vi "Read Relative Calculation.vi"(8 "error in (no error)":errorcluster, 11 "VISA resource name":refnum<visa-resource-name>) -> (0 "error out":errorcluster, 2 "Rel'd Measurement Data":dbl[][](array[numeric]), 3 "VISA resource name out":refnum<visa-resource-name>)   [LabVIEW 2020, in "Keithley 6517.lvlib"]
doc: "Reads the Rel'd measurement data. \n\nRelative (Rel) nulls an offset or subtracts a baseline reading from present and future readings. When a Rel value is established, subsequent readings will be the difference between the actual input and the Rel value.\n\n<B>Displayed (Rel'ed) Reading = Actual Input - Rel Value</B>\n\n<B>Note:</B>\n(1) Rel'd can be configured using <B>Configure Relative Calculation</B> VI.\n(2)This VI is ONLY compatible with <B>model 6514</B>. Running this VI with any other model will result in an error."
uses:
  <instrlib>/Keithley 6517/Keithley 6517.lvlib
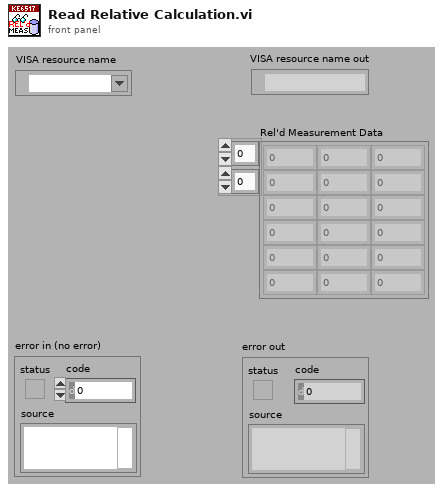
[diagram p1: front panel]
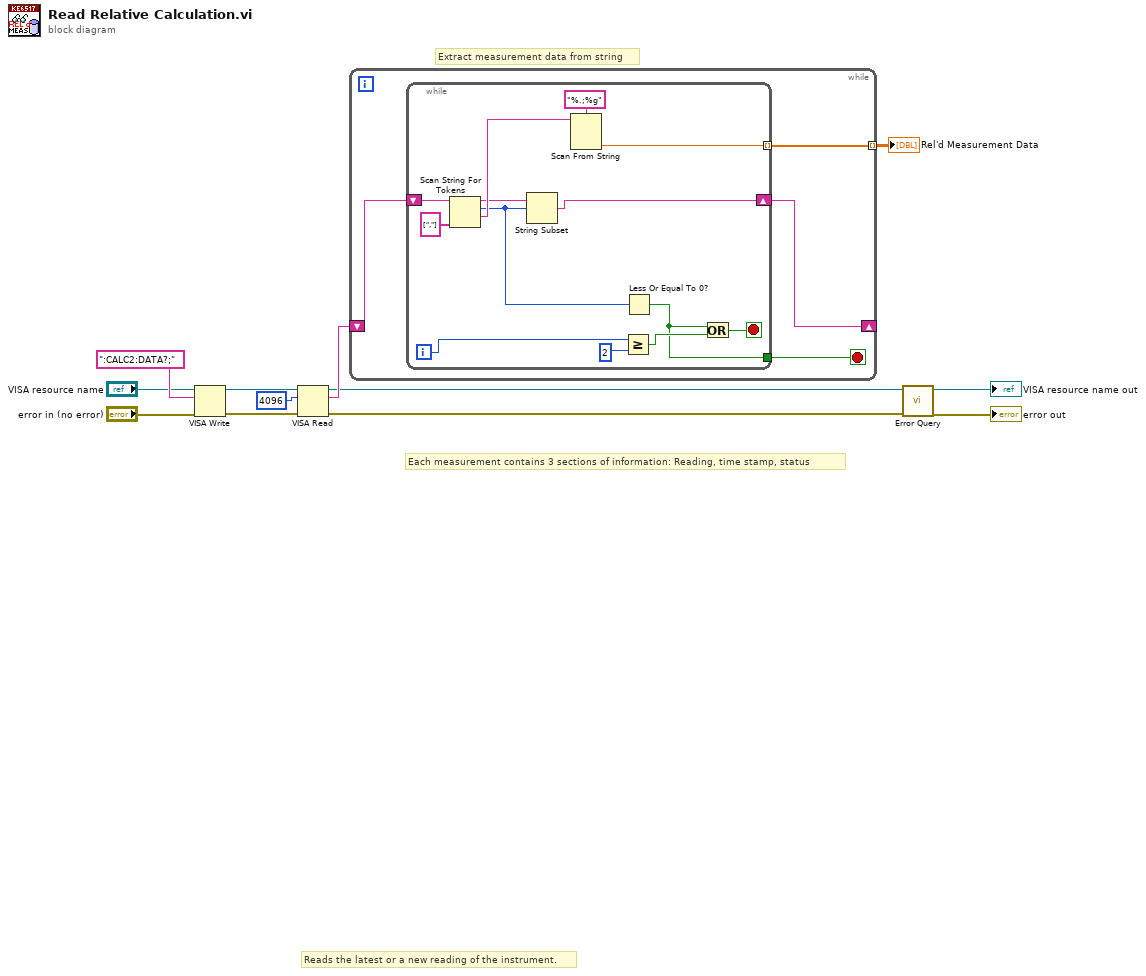
[diagram p0: block diagram]
diagram:
  # "Extract measurement data from string"
  # "Each measurement contains 3 sections of information: Reading, time stamp, status"
  # "Reads the latest or a new reading of the instrument."
  n1 = VISA Write(VISA resource name="VISA resource name", write buffer=":CALC2:DATA?;", error in (no error)="error in (no error)") -> (VISA resource name out=w11:refnum<visa-resource-name>, error out=w10:errorcluster)  [unwired: 1 out]
  n2 = VISA Read(VISA resource name=w11, byte count=u32 4096, error in (no error)=w10) -> (VISA resource name out=w2:refnum<visa-resource-name>, read buffer=w4:string, error out=w1:errorcluster)  [unwired: 1 out]
  n3 = while {
    shift-right: [w15] -> _
    shift-left: w4 -> [w16]
    tunnel: [w13] -> w3 mode=indexing
    stop <- w14 stop-if-true
    n4 = while {
      shift-right: [w21] -> w15
      shift-left: w16 -> [w28]
      tunnel: [w19] -> w14
      tunnel: [w17] -> w13 mode=indexing
      i -> [w18]
      stop <- w23 stop-if-true
      n5 = Scan String For Tokens(6:string[] [","] ("delimiters (\\s,\\t,\\r,\\n)"), 9:w28) -> (1:w27:string, 2:w20:i32, 3:w24:string)  [unwired: 4 in, 1 out]
      n6 = String Subset(string=w24, offset (0)=w20) -> (substring=w21:string)  [unwired: 1 in]
      n7 = Scan From String(format string="%.;%g", input string=w27) -> (output 1=w17:dbl)  [unwired: 3 in, 3 out]
      n8 = Greater Or Equal?(x=w18, y=2) -> (x >= y?=w22:bool)
      n9 = Less Or Equal To 0?(x=w20) -> (x <= 0?=w19:bool)
      n10 = Or(x=w19, y=w22) -> (x .or. y?=w23:bool)
    }
  }
  "Rel'd Measurement Data" <- w3
  n11 = call <instrlib>:"Error Query.vi"("error in (no error)"=w1, "VISA resource name"=w2) -> ("error out"=→"error out":errorcluster, "VISA resource name out"=→"VISA resource name out":refnum<visa-resource-name>)  [unwired: 6 in, 2 out]
